vi "Close Log File.vi"(8 "error in (no error)":errorcluster, 11 "Log File":refnum<k34>) -> (0 "error out":errorcluster)   [LabVIEW 2015]
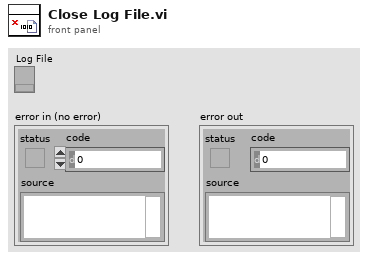
[diagram p1: front panel]
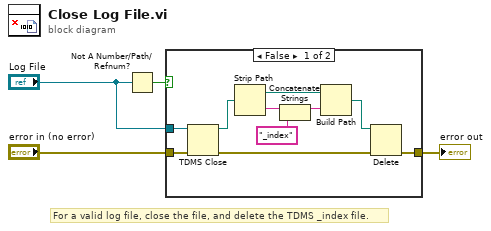
[diagram p0: block diagram]
diagram:
  # "For a valid log file, close the file, and delete the TDMS _index file."
  n1 = Not A Number/Path/Refnum?(number/path/refnum="Log File") -> (NaN/Path/Refnum?=w1:bool)
  n2 = case shown="False" w1 {
    tunnel: [w13 w15] -> w4
    tunnel: "error in (no error)" -> [w6 w15]
    tunnel: "Log File" -> [w5 _]
    frame False {
      n3 = TDMS Close(8:w6, 11:w5) -> (0:w7:errorcluster, 3:w8:path)
      n4 = Strip Path(path=w8) -> (stripped path=w11:path, name=w9:string)
      n5 = Concatenate Strings(w9, "_index") -> (w12:string)
      n6 = Build Path(base path=w11, name or relative path=w12) -> (appended path=w14:path)
      n7 = Delete(path (use dialog)=w14, error in=w7) -> (error out=w13:errorcluster)  [unwired: 3 in, 2 out]
    }
    frame True {
    }
  }
  "error out" <- w4
